vi "FTW-Test-JSON-Stress.vi"() -> (0 "Test Result":errorcluster)   [LabVIEW 2014]
uses:
  src/error/FTW-ERR-Assert-DeveloperError.vi
  src/error/FTW-ERR-ThrowError.vi
  src/error/FTW-ERR-CallChain.vi
  src/string/FTW-STR-ReplaceWhitespace.vi
panel:
  out "Serialized JSON":string[](array[string])
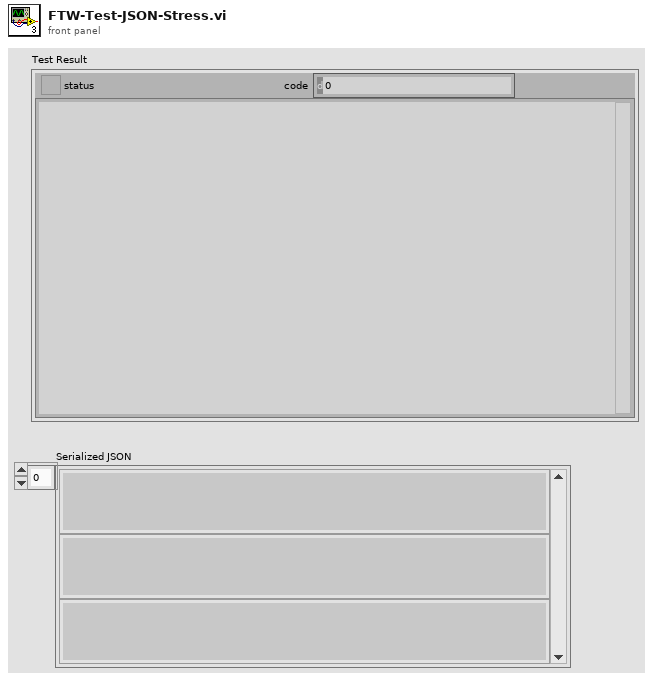
[diagram p1: front panel]
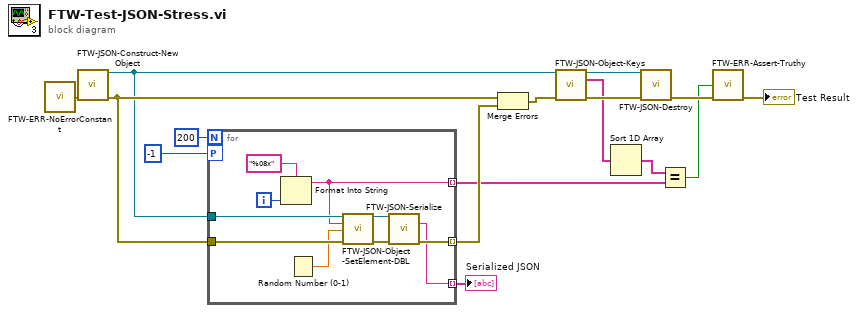
[diagram p0: block diagram]
diagram:
  n1 = call "FTW-ERR-NoErrorConstant.vi"() -> ("no error"=w5:errorcluster)
  n2 = call "FTW-JSON-Construct-NewObject.vi"("error in"=w5) -> ("JSON Object"=w13:refnum<data-value>, "error out"=w14:errorcluster)  [unwired: 13 in]
  n3 = for {
    N: 200 -> [_]
    tunnel: [w22] -> w2 mode=indexing
    workers-P: -1 -> [_]
    tunnel: w14 -> [w25]
    tunnel: [w24] -> w15 mode=indexing
    tunnel: w13 -> [w26]
    tunnel: [w17] -> w11 mode=indexing
    i -> [w18]
    n4 = Format Into String(format string="%08x", w18) -> (resulting string=w17:string)  [unwired: 2 in, 1 out]
    n5 = Random Number (0-1)() -> (number: 0 to 1=w23:dbl)
    n6 = call "FTW-JSON-Object-SetElement-DBL.vi"("JSON Object"=w26, "Key"=w17, "Value"=w23, "error in"=w25) -> ("JSON Object out"=w21:refnum<data-value>, "error out"=w20:errorcluster)  [unwired: 10 in]
    n7 = call "FTW-JSON-Serialize.vi"("JSON Object"=w21, "error in"=w20) -> ("JSON String (UTF-8)"=w22:string, "error out"=w24:errorcluster)  [unwired: 11 in, 1 out]
  }
  "Serialized JSON" <- w2
  n8 = Merge Errors(w14, w15) -> (w12:errorcluster)
  n9 = call "FTW-JSON-Object-Keys.vi"("JSON Object"=w13, "error in"=w12) -> ("JSON Object out"=w10:refnum<data-value>, "Keys"=w4:string[], "error out"=w9:errorcluster)  [unwired: 11 in]
  n10 = Sort 1D Array(array=w4) -> (sorted array=w3:string[])
  n11 = call "FTW-JSON-Destroy.vi"("JSON Object"=w10, "error in"=w9) -> ("error out"=w8:errorcluster)  [unwired: 13 in]
  n12 = Equal?(x=w3, y=w11) -> (x = y?=w7:bool)
  n13 = call "FTW-ERR-Assert-Truthy.vi"("Expected Truthy"=w7, "error in"=w8) -> ("error out"=→"Test Result":errorcluster)  [unwired: 13 in]
